vi "WaitStop.vi"(8 "error in (no error)":errorcluster, 11 "VISA resource name":refnum<visa-resource-name>) -> (0 "error out":errorcluster)   [LabVIEW 2012, in "ESP300.lvlib"]
doc: "Performs an instrument error query before terminating the software connection to the instrument."
uses:
  <instrlib>/ESP300/ESP300.lvlib
  <instrlib>/ESP300/Public/Position_ESP300.vi
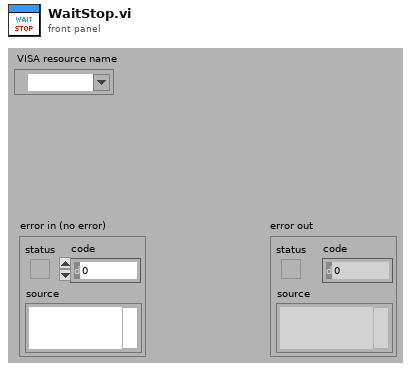
[diagram p1: front panel]
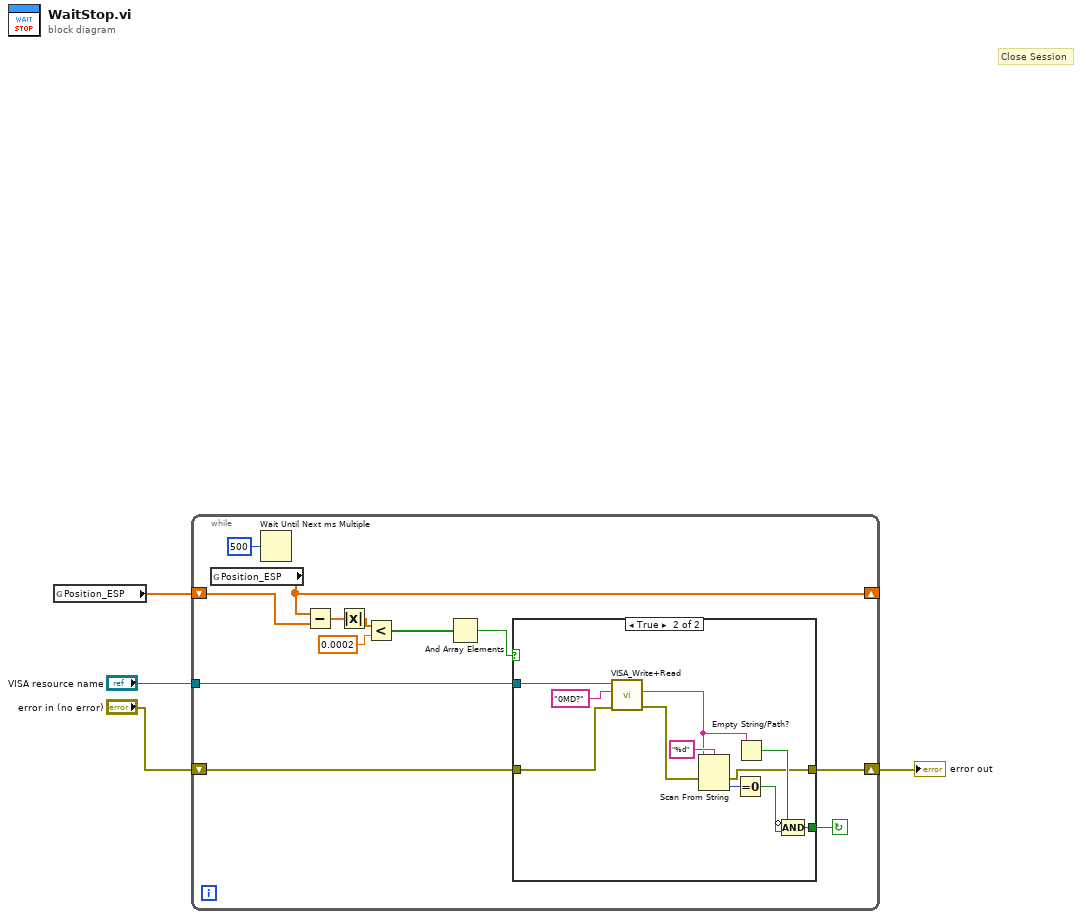
[diagram p0: block diagram]
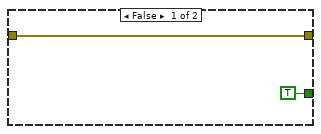
[diagram p2: hidden frame]
diagram:
  # "Close Session"
  n1 = global read "Position_ESP300.vi" "Position_ESP"() -> (w1:dbl[])
  n2 = while {
    tunnel: "VISA resource name" -> [w16]
    shift-right: [w15] -> w3
    shift-left: "error in (no error)" -> [w14]
    shift-right: [w11] -> _
    shift-left: w1 -> [w10]
    stop <- w13 continue-if-true
    n3 = global read "Position_ESP300.vi" "Position_ESP"() -> (w11:dbl[])
    n4 = Wait Until Next ms Multiple(millisecond multiple=u32 500) -> ()  [unwired: 1 out]
    n5 = Subtract(x=w11, y=w10) -> (x-y=w8:dbl[])
    n6 = Absolute Value(x=w8) -> (abs(x)=w5:dbl[])
    n7 = Less?(x=w5, y=0.0002) -> (x < y?=w6:bool[])
    n8 = And Array Elements(Boolean array=w6) -> (logical AND=w9:bool)
    n9 = case shown="True" w9 {
      tunnel: w16 -> [_ w22]
      tunnel: [w18 w21] -> w15
      tunnel: w14 -> [w18 w20]
      tunnel: [TRUE w19] -> w13
      frame False {
      }
      frame True {
        n10 = call <instrlib>:"VISA_Write+Read.vi"("error in (no error)"=w20, "Write Buffer"="0MD?" ("string"), "VISA resource name"=w22) -> ("error out"=w23:errorcluster, "readout"=w25:string)  [unwired: 6 in, 1 out]
        n11 = Scan From String(format string="%d", input string=w25, error in=w23) -> (error out=w21:errorcluster, output 1=w29:i32)  [unwired: 2 in, 2 out]
        n12 = Equal To 0?(x=w29) -> (x = 0?=w26:bool)
        n13 = Empty String/Path?(string/path=w25) -> (empty?=w24:bool)
        n14 = Compound Arithmetic op=AND(invert w24, w26) -> (w19:bool)
      }
    }
  }
  "error out" <- w3
